vi "Cells pos Write.vi"(4 "error in (no error)":errorcluster, 5 "Value":dbl[](array[numeric]), 6 "Container State":T3, 7 "Display State In":T1={"param"={"Short"={"min"=-100.0, "max"=48.0, "real pos"=-48.0}, "Long"={"min"=-900.0, "max"=100.0, "real pos"=-100.0}}, "pos short"=0.0, "pos long"=0.0, "DL short"=refnum, "DL long"=refnum, "Cells"=enum."7", "cell pos"=[], "step,ps"=100}) -> (0 "error out":errorcluster, 3 "Display State Out":T1={"param"={"Short"={"min"=-100.0, "max"=48.0, "real pos"=-48.0}, "Long"={"min"=-900.0, "max"=100.0, "real pos"=-100.0}}, "pos short"=0.0, "pos long"=0.0, "DL short"=refnum, "DL long"=refnum, "Cells"=enum."7", "cell pos"=[], "step,ps"=100})   [LabVIEW 2018, in "ControlDL.xctl"]
uses:
  ControlDL.xctl
  <vilib>/_xctls/Container State.ctl
  stateDL.ctl
  controls/CellsSD.ctl
  controls/CellBoolean.ctl
  <vilib>/_xctls/XControlSupport.lvlib
panel:
  # "Replace the Value Control below with a Control of desired type.\nDo not remove this Control or the others from the connector pane.\nDo not change the connector pane pattern.\nThe Value control should always be the third terminal from top on the input side in the connector pane."
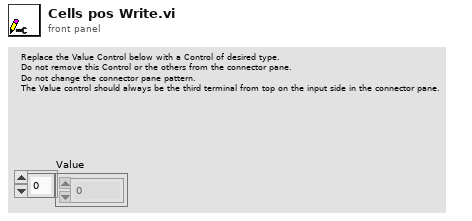
[diagram p1: front panel]
types:
  T1 = typedef "ControlDL.xctl/stateDL.ctl" = cluster{"param":cluster{"Short":cluster{"min":dbl, "max":dbl, "real pos":dbl}, "Long":cluster{"min":dbl, "max":dbl, "real pos":dbl}}, "pos short":dbl, "pos long":dbl, "DL short":refnum<user-event>, "DL long":refnum<user-event>, "Cells":T2, "cell pos":dbl[], "step,ps":i32}
  T2 = typedef "CellsSD.ctl" = enum32{"7", "6", "5", "4", "3", "2", "1", "L"}
  T3 = typedef "XControlSupport.lvlib/Container State.ctl" = cluster{"Indicator?":bool, "Run Mode?":bool, " Refnum":refnum<vi>}
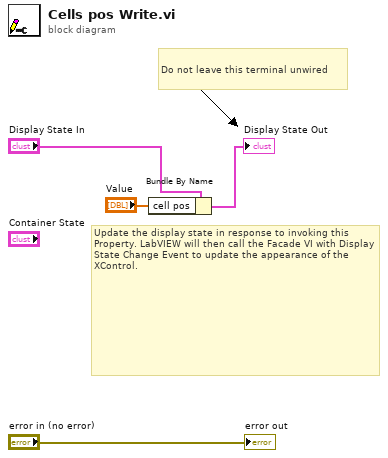
[diagram p0: block diagram]
diagram:
  # "Do not leave this terminal unwired"
  # "Update the display state in response to invoking this Property. LabVIEW will then call the Facade VI with Display State Change Event to update the appearance of the XControl."
  n1 = Bundle By Name(cluster="Display State In", "cell pos"="Value") -> (→"Display State Out":T1)
  "error out" <- "error in (no error)"
